vi "Render Copy.vi"(6 "Destination Rectangle Pointer":u32 format="%.0x", 8 "error in":errorcluster, 9 "Source Rectangle Pointer":u32 format="%.0x", 10 "Texture Pointer":u32 format="%.0x", 11 "Renderer Pointer":u32 format="%.0x") -> (0 "error out":errorcluster, 3 "Return":i32)   [LabVIEW 2014, in "LibSDL2.lvlib"]
uses:
  LibSDL2.lvlib
  DLL/SDL2.dll
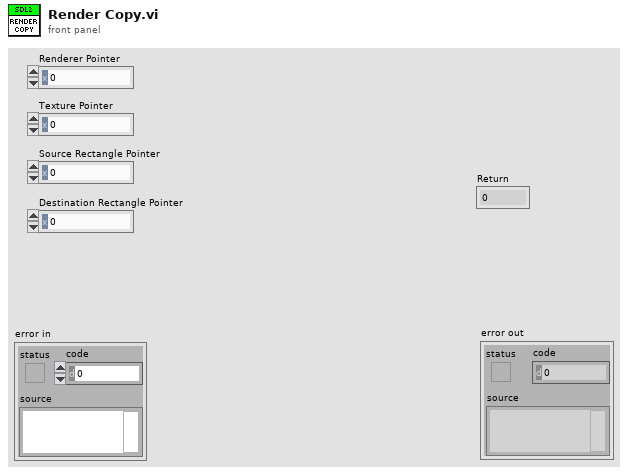
[diagram p1: front panel]
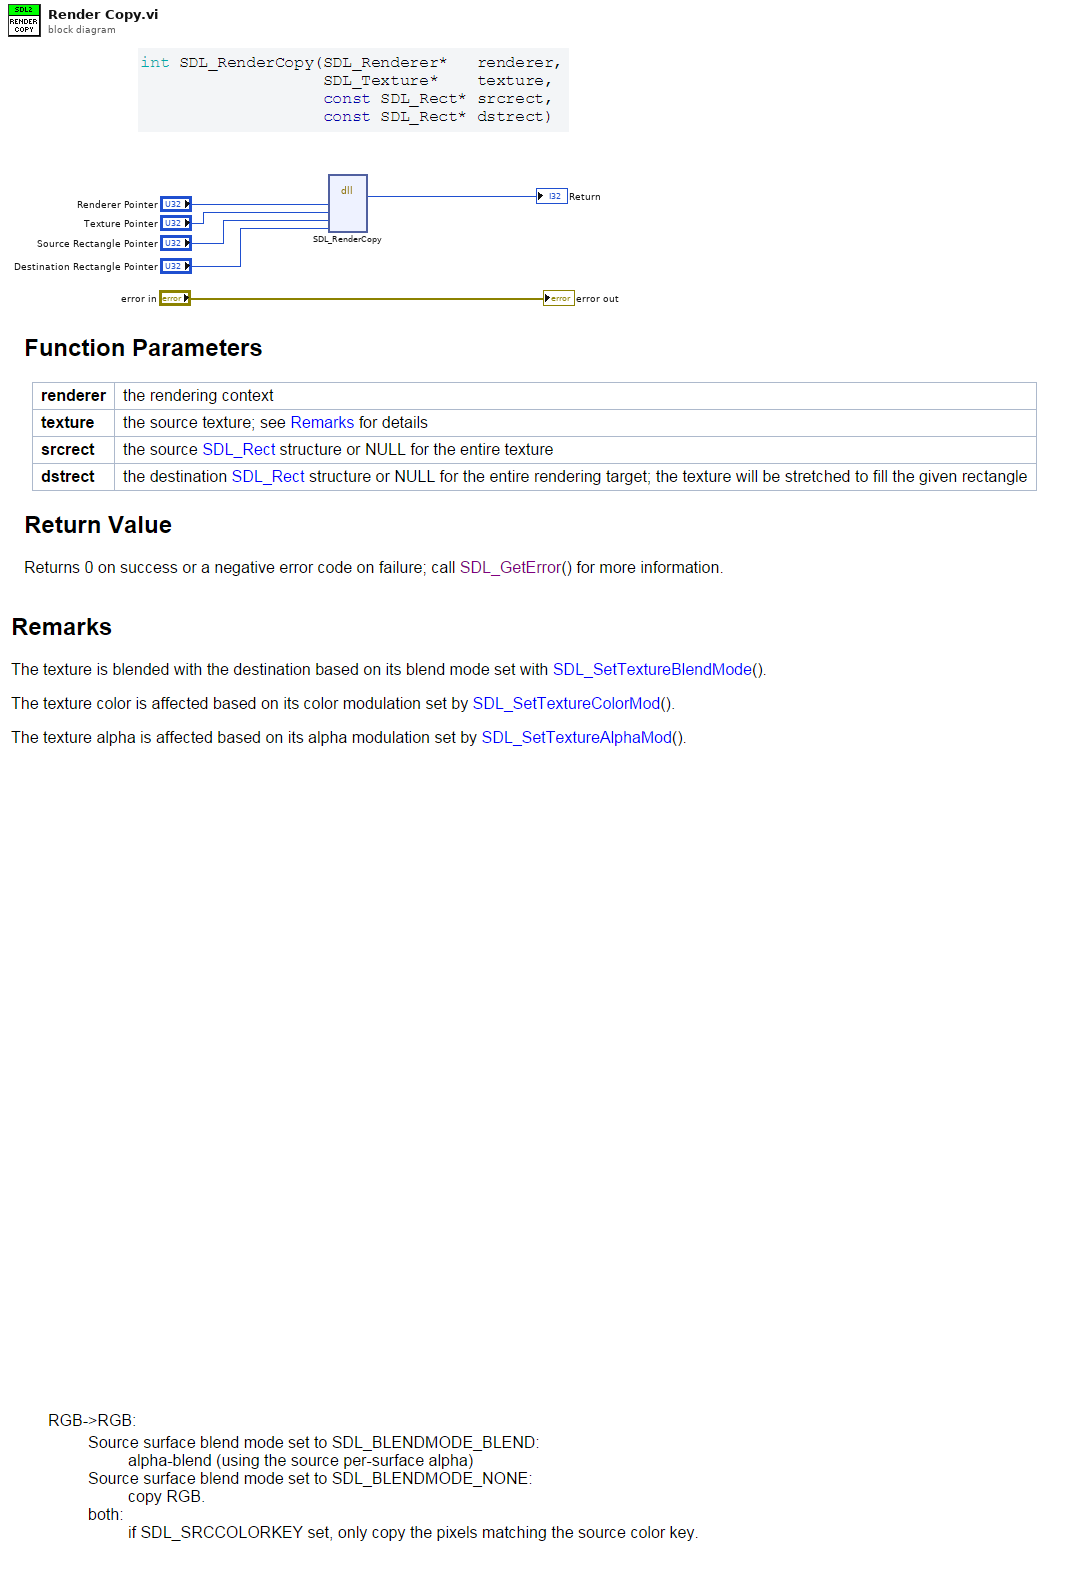
[diagram p0: block diagram]
diagram:
  n1 = dll-call lib="C:/dev/PGS/LabSDL2/Source/LibSDL2 Wrapper/DLL/SDL2.dll" fn="SDL_RenderCopy"("renderer_pointer"="Renderer Pointer", "texture_pointer"="Texture Pointer", "srcrect_pointer"="Source Rectangle Pointer", "dstrect_pointer"="Destination Rectangle Pointer") -> ("return type"=→"Return":i32)  [unwired: 7 in, 2 out]
  "error out" <- "error in"
